vi "Sort Controls.vi"(11 "cluster ref":refnum<vi>) -> (2 "AI controls":refnum<vi>[](array[refnum]), 3 "AO controls":refnum<vi>[](array[refnum]))   [LabVIEW 2020, in "PXISlot.xctl"]
uses:
  PXISlot.xctl
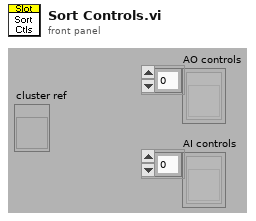
[diagram p1: front panel]
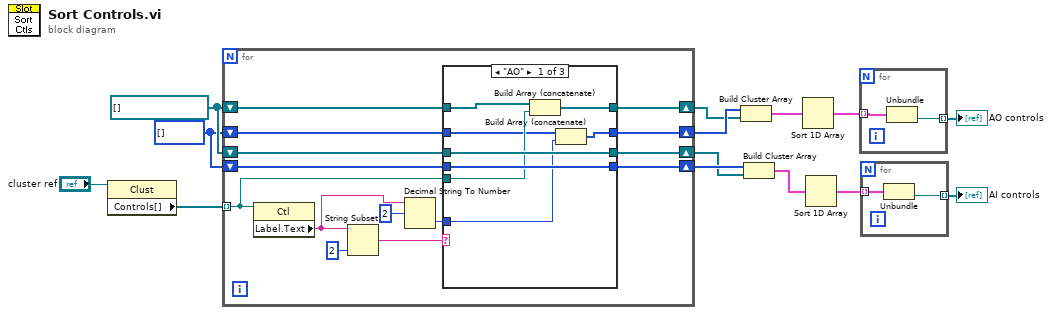
[diagram p0: block diagram]
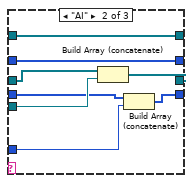
[diagram p2: hidden frame]
diagram:
  w12 = i32[] []
  w13 = refnum<vi>[] [] ("Controls[]")
  n1 = property class="Clust"(reference="cluster ref") -> ("Controls[]"=w14:refnum<vi>[])  [unwired: 1 in, 2 out]
  n2 = for {
    tunnel: w14 -> [w19] mode=indexing
    shift-right: [w22] -> w11
    shift-left: w12 -> [w26]
    shift-right: [w23] -> w10
    shift-left: w13 -> [w27]
    shift-right: [w21] -> w4
    shift-left: w13 -> [w25]
    shift-right: [w20] -> w5
    shift-left: w12 -> [w24]
    n3 = property class="Ctl"(reference=w19) -> ("Label.Text"=w18:string)  [unwired: 1 in, 2 out]
    n4 = String Subset(string=w18, length (rest)=2 ("length (rest)")) -> (substring=w15:string)  [unwired: 1 in]
    n5 = Decimal String To Number(string=w18, offset=2 ("offset (0)")) -> (number=w16:i32)  [unwired: 1 in, 1 out]
    n6 = case shown="\"AO\"" w15 {
      tunnel: w27 -> [w34 w44 w48]
      tunnel: w26 -> [w31 w43 w47]
      tunnel: w25 -> [w36 w40 w46]
      tunnel: w24 -> [w35 w39 w45]
      tunnel: [w32 w44 w48] -> w23
      tunnel: [w30 w43 w47] -> w22
      tunnel: [w36 w42 w46] -> w21
      tunnel: [w35 w38 w45] -> w20
      tunnel: w19 -> [w33 w41 _]
      tunnel: w16 -> [w29 w37 _]
      frame "AO" {
        n7 = Build Array (concatenate)(w34, w33) -> (w32:refnum<vi>[])
        n8 = Build Array (concatenate)(w31, w29) -> (w30:i32[])
      }
      frame "AI" {
        n9 = Build Array (concatenate)(w40, w41) -> (w42:refnum<vi>[])
        n10 = Build Array (concatenate)(w39, w37) -> (w38:i32[])
      }
      frame "", Default {
      }
    }
  }
  n11 = Build Cluster Array(w11, w10) -> (w9:cluster{i32, refnum<vi>}[])
  n12 = Build Cluster Array(w5, w4) -> (w3:cluster{i32, refnum<vi>}[])
  n13 = Sort 1D Array(array=w9) -> (sorted array=w8:cluster{i32, refnum<vi>}[])
  n14 = Sort 1D Array(array=w3) -> (sorted array=w2:cluster{i32, refnum<vi>}[])
  n15 = for {
    tunnel: w8 -> [w50] mode=indexing
    tunnel: [w49] -> w7 mode=indexing
    n16 = Unbundle(w50) -> (w49:refnum<vi>)  [unwired: 1 out]
  }
  "AO controls" <- w7
  n17 = for {
    tunnel: w2 -> [w52] mode=indexing
    tunnel: [w51] -> w1 mode=indexing
    n18 = Unbundle(w52) -> (w51:refnum<vi>)  [unwired: 1 out]
  }
  "AI controls" <- w1
